vi "FlipBit(U32).vi"(8 "error in (no error)":errorcluster caption="错误输入（无错误）", 10 "Bit(0-31)":u8, 11 "Input(32)":u32 format="%.0x") -> (0 "error out":errorcluster caption="错误输出", 3 "Output(U32)":u32 format="%.0x")   [LabVIEW 2012]
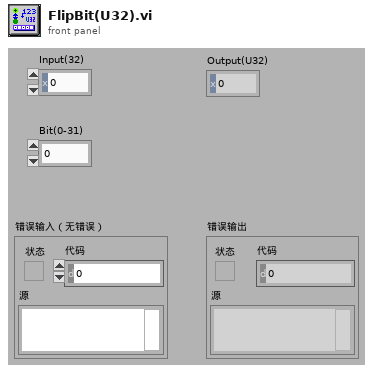
[diagram p1: front panel]
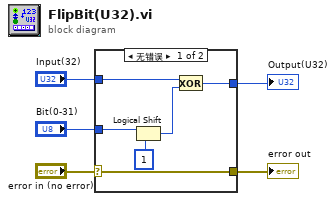
[diagram p0: block diagram]
diagram:
  n1 = case shown="无错误" "error in (no error)" {
    selector: "error in (no error)" -> [w11 w12]
    tunnel: [w11 w12] -> w4
    tunnel: "Bit(0-31)" -> [w9 _]
    tunnel: "Input(32)" -> [w8 _]
    tunnel: [w6 _] -> w1
    frame No Error {
      n2 = Logical Shift(y=w9, x=u32 1) -> (x << y=w7:u32)
      n3 = Exclusive Or(1:w7, 2:w8) -> (0:w6:u32)
    }
    frame Error {
    }
  }
  "error out" <- w4
  "Output(U32)" <- w1
